vi "Open File.vi"(7 "file mode":T1=enum."create/replace", 8 "error in (no error)":errorcluster, 11 "Shared Memory in":refnum<class "Shared Memory.lvclass">) -> (0 "error out":errorcluster, 3 "Shared Memory out":refnum<class "Shared Memory.lvclass">)   [LabVIEW 2013, in "Linux RT IPC.Shared Memory.lvlib" / "Shared Memory.lvclass"]
uses:
  Shared Memory.lvclass
  Controls/file mode.ctl
  Shared Memory.lvclass/Shared Memory.ctl
  C/Controls/file creation flags.ctl
  C/SubVIs/permission group to mode_t.vi
  C/SubVIs/OR flags U32.vi
  C/SubVIs/path globals.vi
  C/SubVIs/error handler.vi
  <vilib>/NI/NI Linux RT Errno/VIs/Public/Get Errno Value for Calling Thread.vi
  C/Linux RT IPC.C.lvlib
  Linux RT IPC.Shared Memory.lvlib
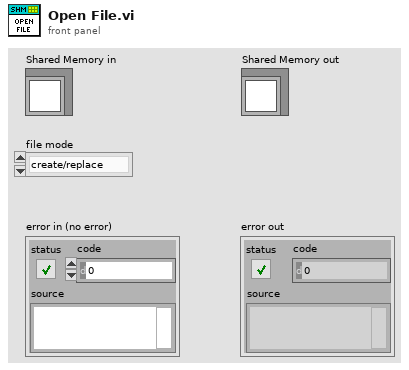
[diagram p1: front panel]
types:
  T1 = typedef "Linux RT IPC.Shared Memory.lvlib/file mode.ctl" = enum16{"open", "create/replace"}
  T2 = typedef "Linux RT IPC.C.lvlib/file creation flags.ctl" = u32
  T3 = cluster{"owner":cluster{"read":bool, "write":bool, "execute":bool}, "group":cluster{"read":bool, "write":bool, "execute":bool}, "everyone":cluster{"read":bool, "write":bool, "execute":bool}}
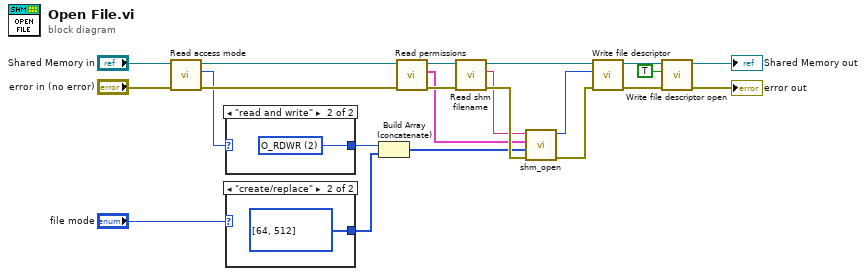
[diagram p0: block diagram]
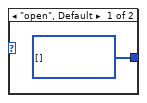
[diagram p2: hidden frame]
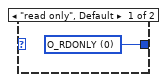
[diagram p3: hidden frame]
diagram:
  n1 = call "Read access mode.vi"("error in (no error)"="error in (no error)", "Shared Memory in"="Shared Memory in") -> ("error out"=w17:errorcluster, "access mode"=w5:enum16{"read only", "read and write"}, "Shared Memory out"=w16:refnum<class "Shared Memory.lvclass">)  [unwired: 7 in]
  n2 = case shown="\"read and write\"" w5 {
    tunnel: [w23 w24] -> w4
    frame "read only", Default {
      w23 = T2 0 items=["O_RDONLY"=0, "O_WRONLY"=1, "O_RDWR"=2, "O_CREAT"=64, "O_EXCL"=128, "O_TRUNC"=512] ("fcntl")
    }
    frame "read and write" {
      w24 = T2 2 items=["O_RDONLY"=0, "O_WRONLY"=1, "O_RDWR"=2, "O_CREAT"=64, "O_EXCL"=128, "O_TRUNC"=512] ("fcntl")
    }
  }
  n3 = case shown="\"create/replace\"" "file mode" {
    tunnel: [w25 w26] -> w2
    frame "open", Default {
      w25 = T2[] [] items=["O_RDONLY"=0, "O_WRONLY"=1, "O_RDWR"=2, "O_CREAT"=64, "O_EXCL"=128, "O_TRUNC"=512] ("file creation flags")
    }
    frame "create/replace" {
      w26 = T2[] [64, 512] items=["O_RDONLY"=0, "O_WRONLY"=1, "O_RDWR"=2, "O_CREAT"=64, "O_EXCL"=128, "O_TRUNC"=512] ("file creation flags")
    }
  }
  n4 = Build Array (concatenate)(w4, w2) -> (w1:T2[])
  n5 = call "Read permissions.vi"("error in (no error)"=w17, "Shared Memory in"=w16) -> ("error out"=w14:errorcluster, "permissions"=w6:T3, "Shared Memory out"=w15:refnum<class "Shared Memory.lvclass">)  [unwired: 7 in]
  n6 = call "Read shm filename.vi"("error in (no error)"=w14, "Shared Memory in"=w15) -> ("error out"=w22:errorcluster, "shm filename"=w13:string, "Shared Memory out"=w11:refnum<class "Shared Memory.lvclass">)  [unwired: 7 in]
  n7 = call "shm_open.vi"("error in (no error)"=w22, "file creation flags"=w1, "permissions (0664)"=w6, "shared memory name"=w13) -> ("error out"=w12:errorcluster, "file descriptor"=w10:i32)  [unwired: 6 in]
  n8 = call "Write file descriptor.vi"("error in (no error)"=w12, "file descriptor"=w10, "Shared Memory in"=w11) -> ("error out"=w21:errorcluster, "Shared Memory out"=w20:refnum<class "Shared Memory.lvclass">)  [unwired: 7 in]
  n9 = call "Write file descriptor open.vi"("error in (no error)"=w21, "file descriptor open"=TRUE, "Shared Memory in"=w20) -> ("error out"=→"error out":errorcluster, "Shared Memory out"=→"Shared Memory out":refnum<class "Shared Memory.lvclass">)  [unwired: 7 in]
